vi "XBeeNO.2_RT.vi"() -> ()   [LabVIEW 2015]
uses:
  <vilib>/Instr/_visa.llb/VISA Configure Serial Port (Instr).vi
panel:
  in  "Transmit Data":string="½n¦t°ê»Ú"
  out "Receive Data":string
  in  "XBee Address":u64[](array[numeric])=[5526146529826801] format="%016x"
  in  "stop":bool
  # "XBeeNO.2  0013A20040E317D7"
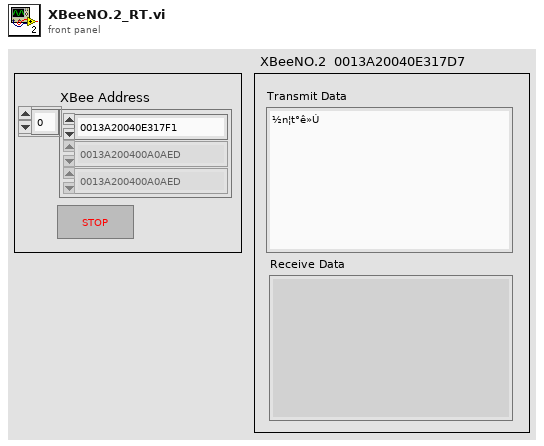
[diagram p1: front panel]
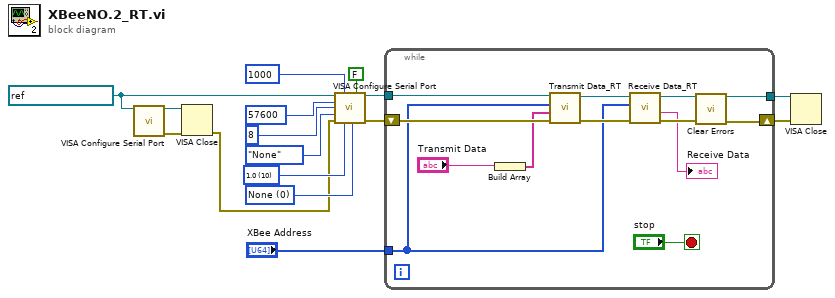
[diagram p0: block diagram]
diagram:
  w2 = refnum<visa-resource-name> "ASRL2::INSTR" ("VISA resource name")
  w13 = u16 10 items=["1.0"=10, "1.5"=15, "2.0"=20] ("stop bits (10: 1 bit)")
  w14 = u16 0 items=["None", "XON/XOFF", "RTS/CTS", "XON/XOFF & RTS/CTS", "DTR/DSR", "XON/XOFF & DTR/DSR"] ("flow control (0:none)")
  n1 = call-poly "VISA Configure Serial Port"("VISA resource name"=w2) -> ("VISA resource name out"=w3:refnum<visa-resource-name>, "error out"=w4:errorcluster)  [unwired: 13 in]
  n2 = VISA Close(VISA resource name=w3, error in (no error)=w4) -> (error out=w1:errorcluster)
  n3 = call-poly "VISA Configure Serial Port"("VISA resource name"=w2, "timeout (10sec)"=u32 1000, "Enable Termination\nChar (T)"=FALSE ("Enable Termination\nChar (T)"), "baud rate (9600)"=u32 57600, "data bits (8)"=u16 8, "parity (0:none)"=enum16{"None", "Odd", "Even", "Mark", "Space"}."None", "error in (no error)"=w1, "stop bits (10: 1 bit)"=w13, "flow control (0:none)"=w14) -> ("VISA resource name out"=w10:refnum<visa-resource-name>, "error out"=w9:errorcluster)  [unwired: 5 in]
  n4 = while {
    tunnel: w10 -> [w23]
    shift-right: [w27] -> w8
    shift-left: w9 -> [w24]
    tunnel: "XBee Address" -> [w20]
    tunnel: [w21] -> w7
    stop <- "stop" stop-if-true
    n5 = Build Array("Transmit Data") -> (w18:string[])
    n6 = call "Transmit Data_RT.vi"("error in (no error)"=w24, "Transmit Data"=w18, "Address"=w20, "VISA resource name"=w23) -> ("error out"=w25:errorcluster, "VISA resource name out"=w26:refnum<visa-resource-name>)  [unwired: 6 in]
    n7 = call "Receive Data_RT.vi"("error in (no error)"=w25, "Address"=w20, "VISA Refnum in"=w26) -> ("error out"=w22:errorcluster, "Receive Data"=→"Receive Data":string, "VISA Refnum out"=w21:refnum<visa-resource-name>)  [unwired: 5 in, 1 out]
    n8 = call <vilib>:"Clear Errors.vi"("error in (no error)"=w22) -> ("error out"=w27:errorcluster)  [unwired: 5 in, 1 out]
  }
  n9 = VISA Close(VISA resource name=w7, error in (no error)=w8) -> ()  [unwired: 1 out]
